vi "Find a Compact Array OD.vi"(8 "error in":errorcluster, 9 "File Refnum":T6, 10 "Index":i32, 11 "ODs":T1[](array[typedef]) {"SubNumber" format="%x"; "AccessType" items=["", "ro", "wo", "rw", "const", "rwr", "rww"]; "DataType" items=[""=0, "BOOLEAN"=1, "INTEGER8"=2, "INTEGER16"=3, "INTEGER32"=4, "UNSIGNED8"=5, "UNSIGNED16"=6, "UNSIGNED32"=7, "REAL32"=8, "VISIBLE_STRING"=9, "OCTET_STRING"=10, "UNICODE_STRING"=11, "TIME_OF_DAY"=12, "TIME_DIFFERENCE"=13, "DOMAIN"=15, "INTEGER24"=16, "REAL64"=17, "INTEGER40"=18, "INTEGER48"=19, "INTEGER56"=20, "INTEGER64"=21, "UNSIGNED24"=22, "UNSIGNED40"=24, "UNSIGNED48"=25, "UNSIGNED56"=26, "UNSIGNED64"=27]; "ObjectType" items=[""=10, "NULL"=0, "DOMAIN"=2, "DEFTYPE"=5, "DEFSTRUCT"=6, "VAR"=7, "ARRAY"=8, "RECORD"=9]; "sub-index" format="%x"; "index" format="%x"}) -> (0 "error out":errorcluster, 1 "Found?":bool, 2 "Next Index":i32, 3 "dup ODs":T1[](array[typedef]) {"SubNumber" format="%x"; "AccessType" items=["", "ro", "wo", "rw", "const", "rwr", "rww"]; "DataType" items=[""=0, "BOOLEAN"=1, "INTEGER8"=2, "INTEGER16"=3, "INTEGER32"=4, "UNSIGNED8"=5, "UNSIGNED16"=6, "UNSIGNED32"=7, "REAL32"=8, "VISIBLE_STRING"=9, "OCTET_STRING"=10, "UNICODE_STRING"=11, "TIME_OF_DAY"=12, "TIME_DIFFERENCE"=13, "DOMAIN"=15, "INTEGER24"=16, "REAL64"=17, "INTEGER40"=18, "INTEGER48"=19, "INTEGER56"=20, "INTEGER64"=21, "UNSIGNED24"=22, "UNSIGNED40"=24, "UNSIGNED48"=25, "UNSIGNED56"=26, "UNSIGNED64"=27]; "ObjectType" items=[""=10, "NULL"=0, "DOMAIN"=2, "DEFTYPE"=5, "DEFSTRUCT"=6, "VAR"=7, "ARRAY"=8, "RECORD"=9]; "sub-index" format="%x"; "index" format="%x"}, 4 "Stop?":bool, 5 "Count":u8)   [LabVIEW 2013]
uses:
  <vilib>/Utility/config.llb/Config Data RefNum.ctl
  control/OD Entry.ctl
  control/Object Type.ctl
  control/Data Type.ctl
  control/Access Type.ctl
  control/OD Cateory.ctl
  <vilib>/Utility/config.llb/NI_LVConfig.lvlib
panel:
  in  "Numeric":u8
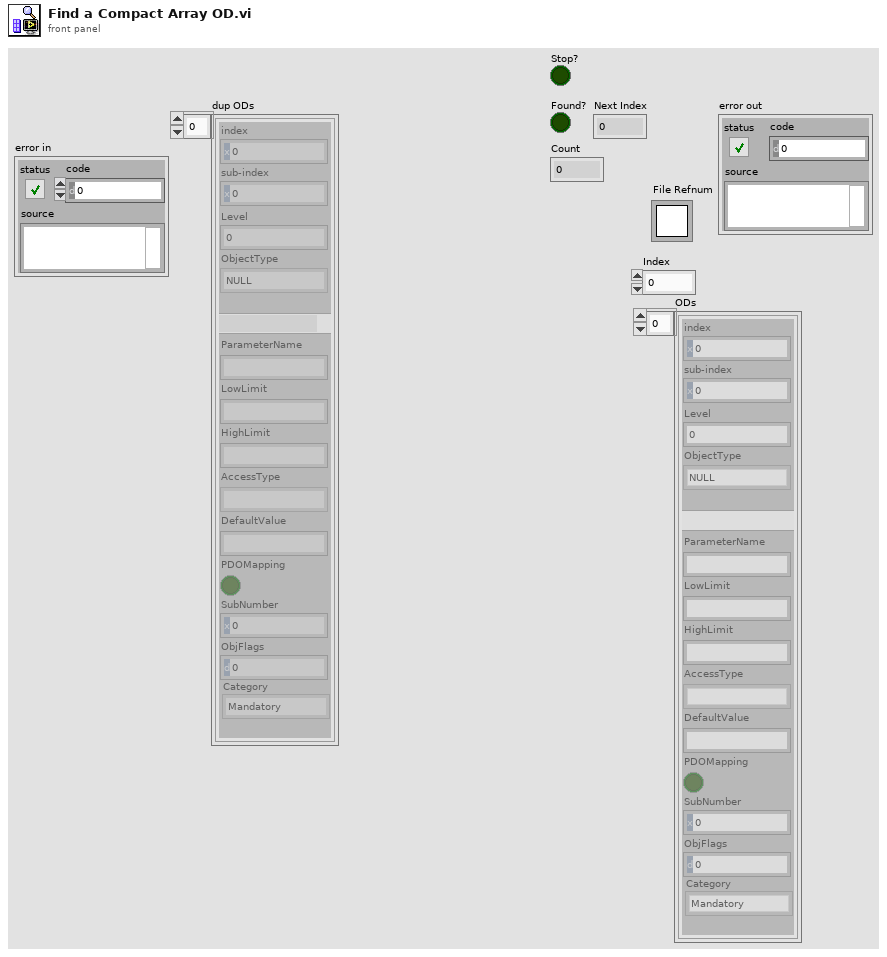
[diagram p1: front panel]
types:
  T1 = typedef "OD Entry.ctl" = cluster{"index":u16, "sub-index":u8, "Level":u8, "ObjectType":T2, "DataType":T3, "ParameterName":string, "LowLimit":string, "HighLimit":string, "AccessType":T4, "DefaultValue":string, "PDOMapping":bool, "SubNumber":u8, "ObjFlags":u32, "Category":T5}
  T2 = typedef "Object Type.ctl" = u16
  T3 = typedef "Data Type.ctl" = u16
  T4 = typedef "Access Type.ctl" = u16
  T5 = typedef "OD Cateory.ctl" = enum16{"Mandatory", "Optional", "Manufacturer", ""}
  T6 = typedef "NI_LVConfig.lvlib/Config Data RefNum.ctl" = refnum<k1>
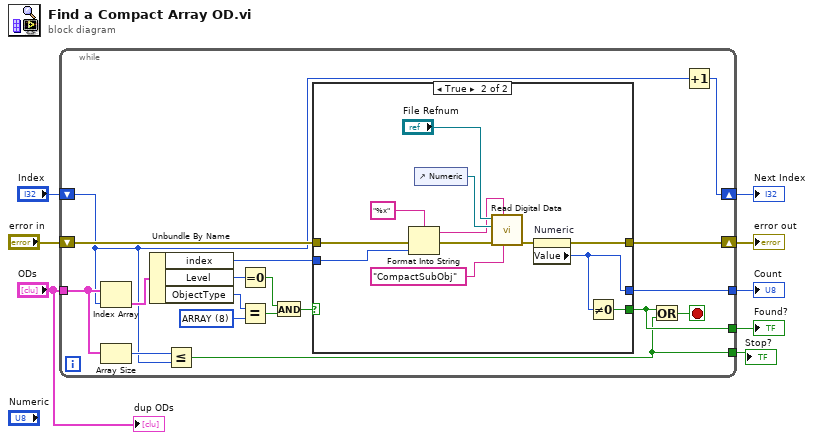
[diagram p0: block diagram]
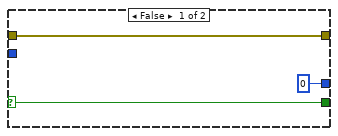
[diagram p2: hidden frame]
diagram:
  n1 = while {
    tunnel: "ODs" -> [w16]
    shift-right: [w19] -> w4
    shift-left: "Index" -> [w15]
    shift-right: [w12] -> w7
    shift-left: "error in" -> [w18]
    tunnel: [w14] -> w5
    tunnel: [w11] -> w3
    tunnel: [w9] -> w1
    stop <- w13 stop-if-true
    w24 = T2 8 items=[""=10, "NULL"=0, "DOMAIN"=2, "DEFTYPE"=5, "DEFSTRUCT"=6, "VAR"=7, "ARRAY"=8, "RECORD"=9] ("y")
    n2 = Index Array(array=w16, index=w15) -> (element=w20:T1)
    n3 = Array Size(array=w16) -> (size(s)=w17:i32)
    n4 = Unbundle By Name(w20) -> ("index"=w10:u16, "Level"=w26:u8, "ObjectType"=w25:T2)
    n5 = Less Or Equal?(x=w17, y=w15) -> (x <= y?=w9:bool)
    n6 = Equal To 0?(x=w26) -> (x = 0?=w23:bool)
    n7 = Equal?(x=w25, y=w24) -> (x = y?=w22:bool)
    n8 = And(x=w23, y=w22) -> (x .and. y?=w21:bool)
    n9 = case shown="True" w21 {
      selector: w21 -> [w29 _]
      tunnel: [w29 w30] -> w14
      tunnel: w18 -> [w28 w39]
      tunnel: [w28 w32] -> w12
      tunnel: [u8 0 ("value") w31] -> w11
      tunnel: w10 -> [_ w41]
      frame False {
      }
      frame True {
        n10 = Format Into String(format string="%x", error in=w39, w41) -> (resulting string=w35:string, error out=w38:errorcluster)  [unwired: 1 in]
        n11 = control-ref of="Numeric"() -> (w36:refnum<vi>)
        n12 = call "Read Digital Data.vi"("Keyword Name"="CompactSubObj" ("key"), "Section Name"=w35, "error in (no error)"=w38, "DigNum Refnum"=w36, "file refnum"="File Refnum") -> ("error out"=w33:errorcluster)  [unwired: 6 in]
        n13 = property on="Numeric" class="DigNum (strict)"(error in=w33) -> (error out=w32:errorcluster, "Value"=w31:u8)  [unwired: 1 in, 1 out]
        n14 = Not Equal To 0?(x=w31) -> (x != 0?=w30:bool)
      }
    }
    n15 = Or(x=w14, y=w9) -> (x .or. y?=w13:bool)
    n16 = Increment(x=w15) -> (x+1=w19:i32)
  }
  "error out" <- w7
  "Found?" <- w5
  "Next Index" <- w4
  "Count" <- w3
  "Stop?" <- w1
  "dup ODs" <- "ODs"
